vi "uTransport_Destroy.vi"(8 "error in (no error)":errorcluster, 11 "uTransport_Queue in":refnum<class "uTransport_Queue.lvclass">) -> (0 "error out":errorcluster)   [LabVIEW 2023, in "uLib.lvlib" / "uTransport_Queue.lvclass"]
uses:
  uTransport_Queue.lvclass
  uTransport_Queue.lvclass/uTransport_Queue.ctl
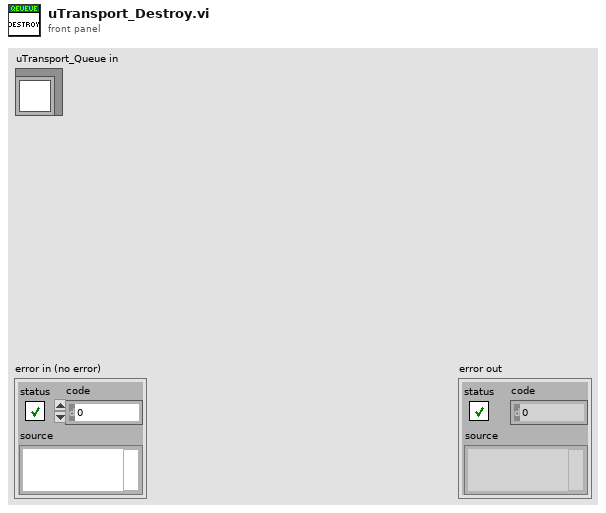
[diagram p1: front panel]
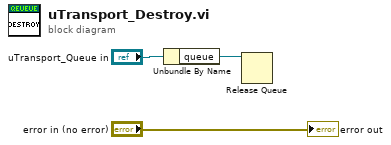
[diagram p0: block diagram]
diagram:
  n1 = Unbundle By Name("uTransport_Queue in") -> ("queue"=w1:refnum<queue>)
  n2 = Release Queue(queue=w1) -> ()  [unwired: 2 in, 3 out]
  "error out" <- "error in (no error)"
